vi "英维克传感器状态解析.vi"(11 "传感器状态输入":u16[](array[numeric])) -> (3 "传感器状态输出":T1)   [LabVIEW 2016, in "环境动力监测库.lvlib" / "空调库.lvlib"]
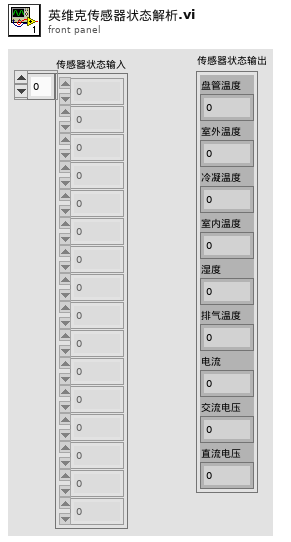
[diagram p1: front panel]
types:
  T1 = cluster{"盘管温度":u16, "室外温度":u16, "冷凝温度":u16, "室内温度":u16, "湿度":u16, "排气温度":u16, "电流":u16, "交流电压":u16, "直流电压":u16}
  T2 = cluster{dbl, dbl, dbl, dbl, dbl, dbl, dbl, dbl, dbl}
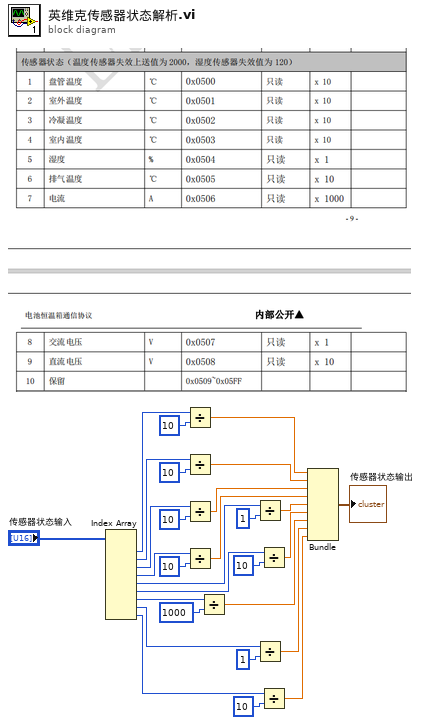
[diagram p0: block diagram]
diagram:
  n1 = Index Array(array="传感器状态输入") -> (element #1=w28:u16, element #2=w26:u16, element #3=w24:u16, element #4=w22:u16, element #5=w20:u16, element #6=w18:u16, element #7=w13:u16, element #8=w12:u16, element #9=w11:u16)  [unwired: 9 in]
  n2 = Divide(x=w28, y=u16 10) -> (x/y=w10:dbl)
  n3 = Divide(x=w26, y=u16 10) -> (x/y=w9:dbl)
  n4 = Divide(x=w24, y=u16 10) -> (x/y=w8:dbl)
  n5 = Divide(x=w22, y=u16 10) -> (x/y=w7:dbl)
  n6 = Divide(x=w13, y=u16 1000) -> (x/y=w3:dbl)
  n7 = Divide(x=w20, y=u16 1) -> (x/y=w5:dbl)
  n8 = Divide(x=w12, y=u16 1) -> (x/y=w2:dbl)
  n9 = Divide(x=w18, y=u16 10) -> (x/y=w4:dbl)
  n10 = Divide(x=w11, y=u16 10) -> (x/y=w1:dbl)
  n11 = Bundle(w10, w9, w8, w7, w5, w4, w3, w2, w1) -> (→"传感器状态输出":T2)  [unwired: 1 in]
